vi "Read BC Subaddress to Buffer ID Map.vi"(8 "error in":errorcluster, 11 "shared resources":refnum<class "Shared Resources.lvclass">) -> (0 "error out":errorcluster, 2 "bc subaddress to buffer id map":T1, 3 "shared resources out":refnum<class "Shared Resources.lvclass">)   [LabVIEW 2020, in "AIM MIL-STD-1553 Engine.lvlib" / "Implementation.lvlib" / "Shared Resources.lvclass"]
uses:
  Shared Resources.lvclass
  BC Subaddress to Buffer ID Map.ctl
  Shared Resources.lvclass/Shared Resources.ctl
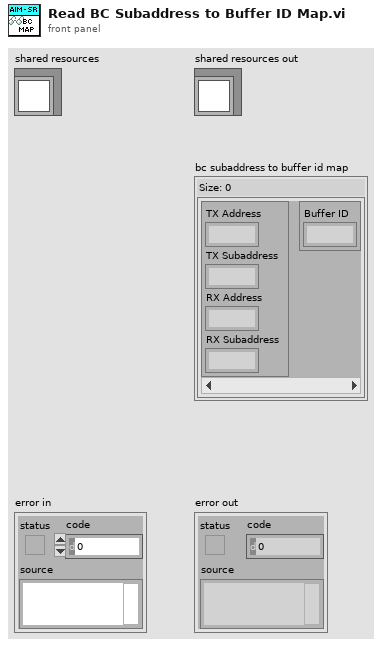
[diagram p1: front panel]
types:
  T1 = typedef "AIM MIL-STD-1553 Engine.lvlib/Implementation.lvlib/Shared Resources.lvclass/BC Subaddress to Buffer ID Map.ctl" = map{cluster{"TX Address":u8, "TX Subaddress":u8, "RX Address":u8, "RX Subaddress":u8}, cluster{"Buffer ID":u16}}
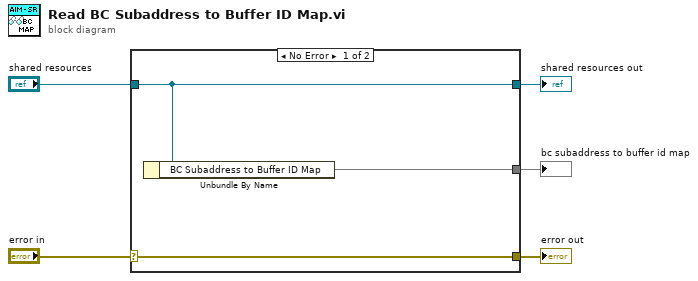
[diagram p0: block diagram]
diagram:
  n1 = case shown="No Error" "error in" {
    selector: "error in" -> [w8 w9]
    tunnel: [w8 w9] -> w4
    tunnel: [w7 w10] -> w2
    tunnel: "shared resources" -> [w7 w10]
    tunnel: [w6 _] -> w1
    frame No Error {
      n2 = Unbundle By Name(w7) -> ("BC Subaddress to Buffer ID Map"=w6:T1)
    }
    frame Error {
    }
  }
  "error out" <- w4
  "shared resources out" <- w2
  "bc subaddress to buffer id map" <- w1
